vi "Assert Excel.vi"() -> ()   [LabVIEW 2015, in "Admin_Actor.lvlib" / "CalAttendance.lvclass"]
uses:
  CalAttendance.lvclass
panel:
  out "data":string[][](array[string])
  in  "path":path
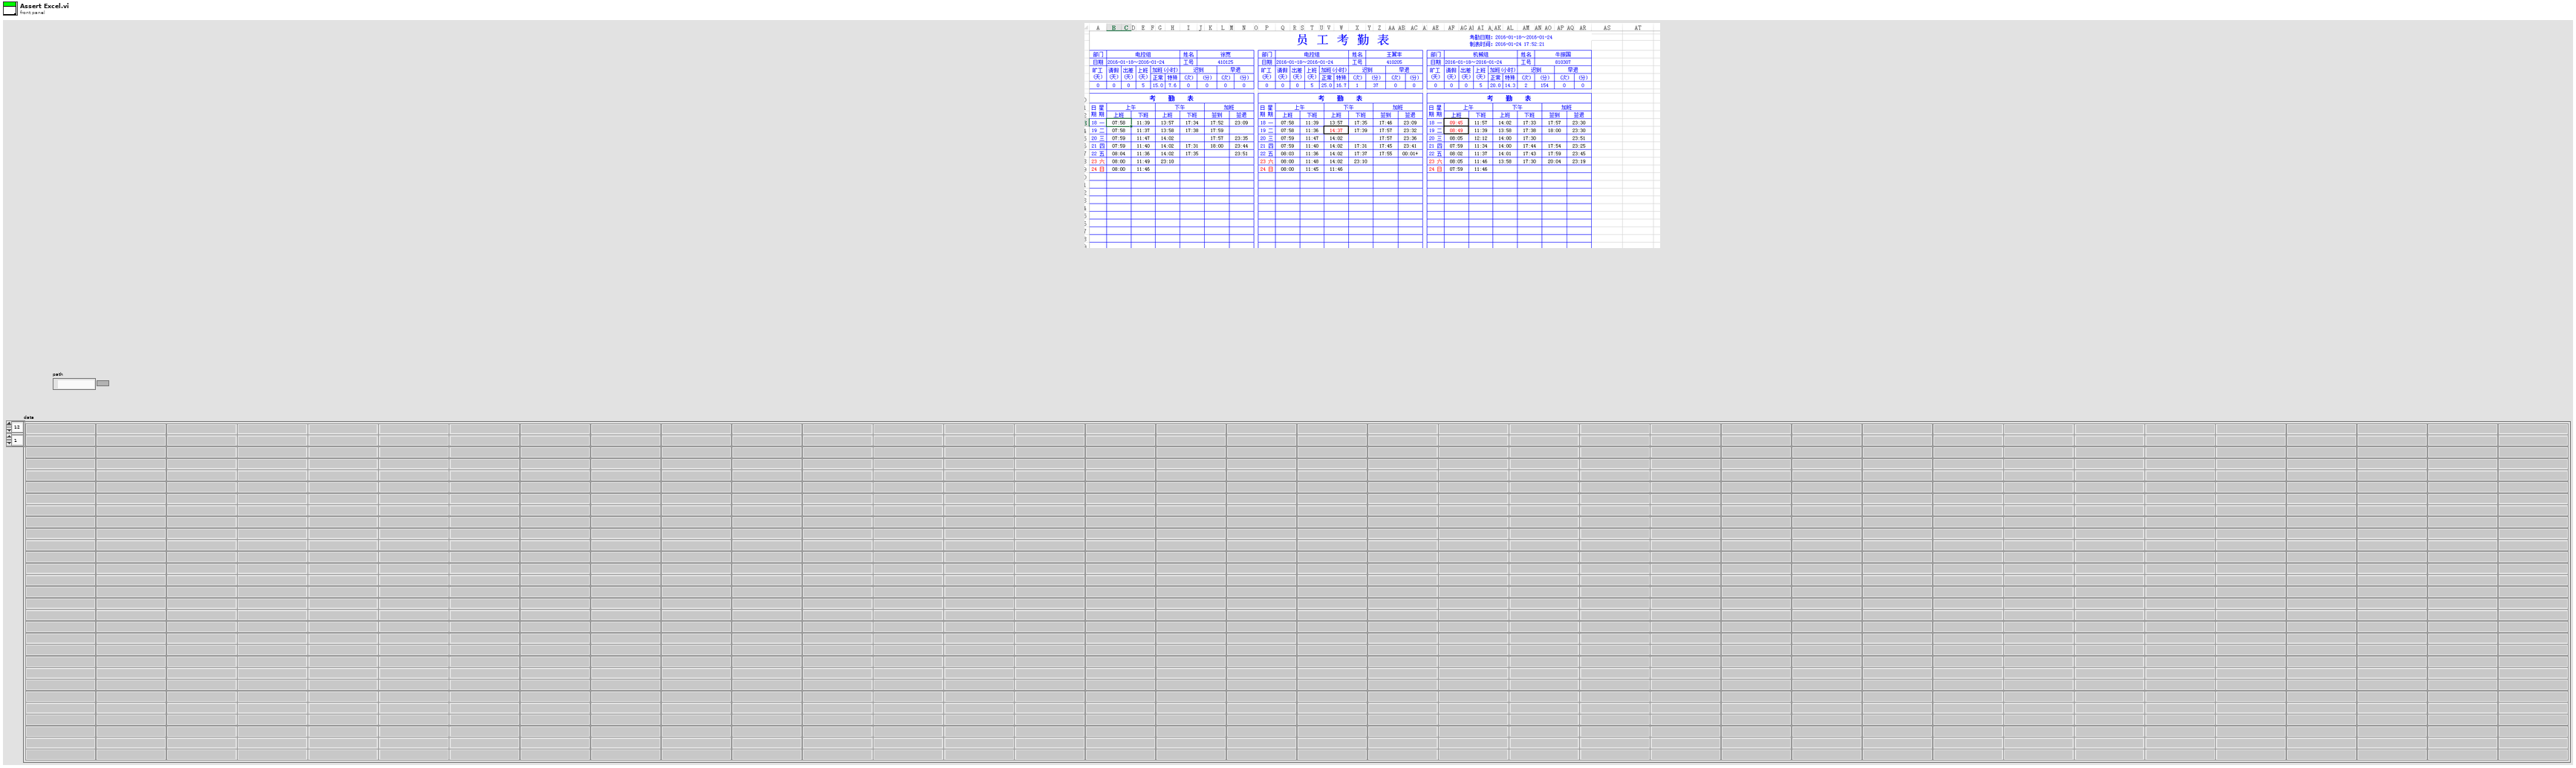
[diagram p1: front panel]
types:
  T1 = cluster{"Excel._Application":refnum<k7>, "Workbooks":refnum<k7>}
  T2 = cluster{"Excel._Application":refnum<k7>, "Workbooks":refnum<k7>, "Open":refnum<k7>}
  T3 = cluster{"Excel._Application":refnum<k7>, "Workbooks":refnum<k7>, "Open":refnum<k7>, "Worksheets":refnum<k7>, "Excel._Worksheet":refnum<k7>}
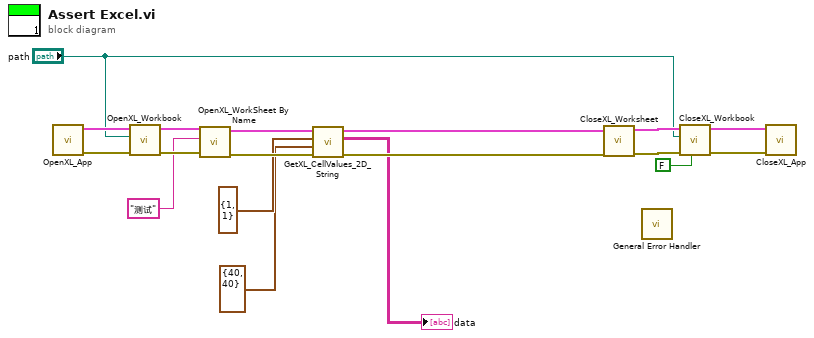
[diagram p0: block diagram]
diagram:
  n1 = call "OpenXL_App.vi"() -> ("error out"=w17:errorcluster, "Refnum Cluster"=w18:T1)  [unwired: 10 in]
  n2 = call "OpenXL_Workbook.vi"("error in"=w17, "path"="path", "Refnum Cluster In"=w18) -> ("error out"=w9:errorcluster, "Refnum Cluster Out"=w10:T2)  [unwired: 7 in]
  n3 = call "OpenXL_WorkSheet By Name.vi"("error in (no error)"=w9, "SheetName(\"\")"="测试" ("SheetName(\"\")"), "Refnum Cluster In"=w10) -> ("error out"=w6:errorcluster, "Refnum Cluster Out"=w7:T3)  [unwired: 7 in]
  n4 = call "GetXL_CellValues_2D_String.vi"("error in"=w6, "End"=cluster{"Column":i32, "Row":i32} {"Column"=40, "Row"=40}, "Start"=cluster{"Column":i32, "Row":i32} {"Column"=1, "Row"=1}, "Refnum Cluster In"=w7) -> ("error out"=w2:errorcluster, "data"=→"data":string[][], "Refnum Cluster Out"=w3:T3)  [unwired: 5 in]
  n5 = call "CloseXL_Worksheet.vi"("error in (no error)"=w2, "Refnum Cluster In"=w3) -> ("error out"=w16:errorcluster, "Refnum Cluster Out"=w15:T2)  [unwired: 8 in]
  n6 = call <vilib>:"General Error Handler.vi"() -> ()  [unwired: 11 in, 5 out]
  n7 = call "CloseXL_Workbook.vi"("Save? (F)"=FALSE, "error in (no error)"=w16, "path"="path", "Refnum Cluster In"=w15) -> ("error out"=w14:errorcluster, "Refnum Cluster Out"=w13:T1)  [unwired: 6 in]
  n8 = call "CloseXL_App.vi"("error in (no error)"=w14, "Refnum Cluster In"=w13) -> ()  [unwired: 9 in, 1 out]
